vi "PEM.vi"(8 "error in (no error)":errorcluster, 9 "Inhibir":bool, 10 "Longitud de Onda":dbl=620.0, 11 "Retardo":i32=500) -> (0 "error out":errorcluster, 2 "Longitud de Onda":dbl, 3 "Retardo":dbl)   [LabVIEW 2018]
uses:
  <vilib>/Instr/_visa.llb/VISA Configure Serial Port (Instr).vi
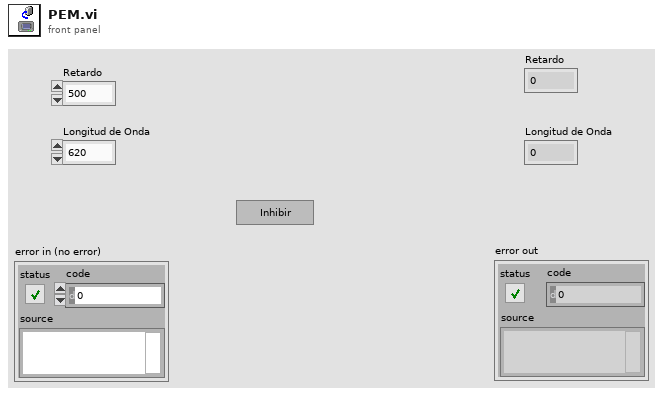
[diagram p1: front panel]
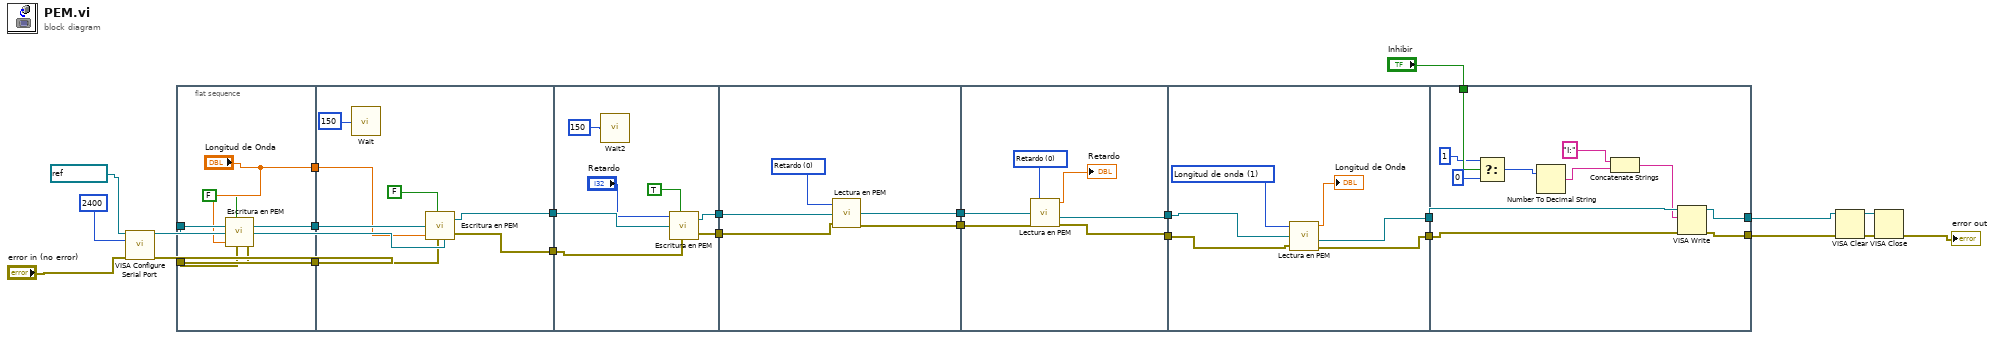
[diagram p0: block diagram]
diagram:
  n1 = call-poly "VISA Configure Serial Port"("VISA resource name"=refnum<visa-resource-name> "COM8", "baud rate (9600)"=u32 2400, "error in (no error)"="error in (no error)") -> ("VISA resource name out"=w16:refnum<visa-resource-name>, "error out"=w21:errorcluster)  [unwired: 11 in]
  n2 = flat-sequence {
    tunnel: w21 -> [w28]
    tunnel: w16 -> [w27]
    tunnel: [w30] -> w7
    tunnel: ["Longitud de Onda"] -> w6
    tunnel: [w29] -> w5
    tunnel: [w34] -> w12
    tunnel: [w32] -> w11
    tunnel: w7 -> [w36]
    tunnel: w6 -> [w31]
    tunnel: w5 -> [w35]
    tunnel: w12 -> [w40]
    tunnel: w11 -> [w43]
    tunnel: [w39] -> w10
    tunnel: [w38] -> w13
    tunnel: w10 -> [w48]
    tunnel: w13 -> [w47]
    tunnel: [w46] -> w9
    tunnel: [w45] -> w14
    tunnel: w9 -> [w54]
    tunnel: w14 -> [w53]
    tunnel: [w51] -> w8
    tunnel: [w50] -> w15
    tunnel: w8 -> [w59]
    tunnel: w15 -> [w58]
    tunnel: [w57] -> w4
    tunnel: [w56] -> w3
    tunnel: [w72] -> w17
    tunnel: w4 -> [w69]
    tunnel: w3 -> [w70]
    tunnel: "Inhibir" -> [w68]
    tunnel: [w71] -> w1
    frame #0 {
      n3 = call "Escritura en PEM.vi"("Retardo"=FALSE, "VISA resource name"=w27, "Longitud de onda nm"="Longitud de Onda", "error in (no error)"=w28) -> ("VISA resource name out"=w30:refnum<visa-resource-name>, "error out"=w29:errorcluster)  [unwired: 1 in]
    }
    frame #1 {
      n4 = call "Wait"("Count(mSec)"=u32 150) -> ()  [unwired: 1 out]
      n5 = call "Escritura en PEM.vi"("Retardo"=FALSE, "VISA resource name"=w36, "Longitud de onda nm"=w31, "error in (no error)"=w35) -> ("VISA resource name out"=w32:refnum<visa-resource-name>, "error out"=w34:errorcluster)  [unwired: 1 in]
    }
    frame #2 {
      n6 = call "Wait2"("Count(mSec)"=u32 150) -> ()  [unwired: 1 out]
      n7 = call "Escritura en PEM.vi"("Retardo de onda lambda"="Retardo", "Retardo"=TRUE, "VISA resource name"=w43, "error in (no error)"=w40) -> ("VISA resource name out"=w39:refnum<visa-resource-name>, "error out"=w38:errorcluster)  [unwired: 1 in]
    }
    frame #3 {
      w49 = u16 0 items=["Retardo", "Longitud de onda", "Frecuencia 1", "Frecuencia 2"] ("Caracteristica a leer")
      n8 = call "Lectura en PEM.vi"("Caracteristica a leer"=w49, "VISA resource name"=w48, "error in (no error)"=w47) -> ("VISA resource name out"=w46:refnum<visa-resource-name>, "error out"=w45:errorcluster)  [unwired: 2 out]
    }
    frame #4 {
      w52 = u16 0 items=["Retardo", "Longitud de onda", "Frecuencia 1", "Frecuencia 2"] ("Caracteristica a leer")
      n9 = call "Lectura en PEM.vi"("Caracteristica a leer"=w52, "VISA resource name"=w54, "error in (no error)"=w53) -> ("Valor leído"=→"Retardo":dbl, "VISA resource name out"=w51:refnum<visa-resource-name>, "error out"=w50:errorcluster)  [unwired: 1 out]
    }
    frame #5 {
      w60 = u16 1 items=["Retardo", "Longitud de onda", "Frecuencia 1", "Frecuencia 2"] ("Caracteristica a leer")
      n10 = call "Lectura en PEM.vi"("Caracteristica a leer"=w60, "VISA resource name"=w59, "error in (no error)"=w58) -> ("Valor leído"=→"Longitud de Onda":dbl, "VISA resource name out"=w56:refnum<visa-resource-name>, "error out"=w57:errorcluster)  [unwired: 1 out]
    }
    frame #6 {
      n11 = Select(t=1, s=w68, f=0) -> (s? t:f=w64:i32)
      n12 = Number To Decimal String(number=w64) -> (decimal integer string=w63:string)  [unwired: 1 in]
      n13 = Concatenate Strings("I:", w63) -> (w62:string)
      n14 = VISA Write(VISA resource name=w70, write buffer=w62, error in (no error)=w69) -> (VISA resource name out=w72:refnum<visa-resource-name>, error out=w71:errorcluster)  [unwired: 1 out]
    }
  }
  n15 = VISA Clear(VISA resource name=w17, error in (no error)=w1) -> (VISA resource name out=w20:refnum<visa-resource-name>, error out=w19:errorcluster)
  n16 = VISA Close(VISA resource name=w20, error in (no error)=w19) -> (error out=→"error out":errorcluster)
